vi "DisconnectFromServer.vi"(4 "Reason":string, 5 "Code":u16=1000, 6 "error in":errorcluster, 9 "connection ID":refnum<k5>) -> (0 "error out":errorcluster)   [LabVIEW 2014, in "Raspberry Pi Compatible Compiler for LabVIEW.lvlib" / "Websocket.lvlib"]
uses:
  Websocket.lvlib
  WebsocketFrameTypes_TD.ctl
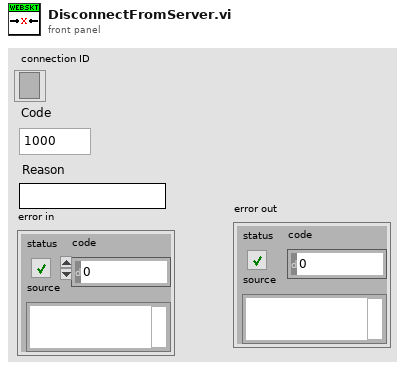
[diagram p1: front panel]
types:
  T1 = typedef "Raspberry Pi Compatible Compiler for LabVIEW.lvlib/Websocket.lvlib/WebsocketFrameTypes_TD.ctl" = enum8{"Continuation", "Text", "Binary", "Reserved 1", "Reserved 2", "Reserved 3", "Reserved 4", "Reserved 5", "Close", "Ping", "Pong", "Reserved 6", "Reserved 7", "Reserved 8", "Reserved 9", "Reserved 10"}
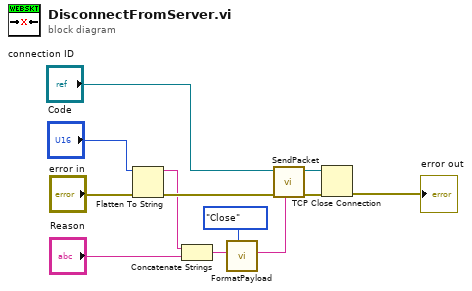
[diagram p0: block diagram]
diagram:
  n1 = Flatten To String(anything="Code", error in (no error)="error in") -> (data string=w7:string, error out=w10:errorcluster)  [unwired: 2 in, 1 out]
  n2 = Concatenate Strings(w7, "Reason") -> (w6:string)
  n3 = call "FormatPayload.vi"("opcode"=WebsocketFrameTypes_TD."Close", "payload"=w6) -> ("packet"=w8:string)  [unwired: 9 in]
  n4 = call "SendPacket.vi"("payload"=w8, "error in"=w10, "connection ID"="connection ID") -> ("error out"=w3:errorcluster, "connection ID out"=w2:refnum<k5>)  [unwired: 5 in]
  n5 = TCP Close Connection(connection ID=w2, error in (no error)=w3) -> (error out=→"error out":errorcluster)  [unwired: 1 in, 1 out]
